vi "Normalized CC IMAQ.vi"(0 "Template U16":T1, 7 "A U16":T1, 11 "Error In":errorcluster) -> (4 "normxcorr2":dbl[][](array[numeric]), 15 "Error Out":errorcluster)   [LabVIEW 2020]
uses:
  <vilib>/vision/Image Controls.llb/IMAQ Image.ctl
  <vilib>/Analysis/2dsp.llb/2D Cross Correlation (CDB).vi
  <vilib>/Analysis/NI_AALPro.lvlib
  <vilib>/Analysis/NI_AALBase.lvlib
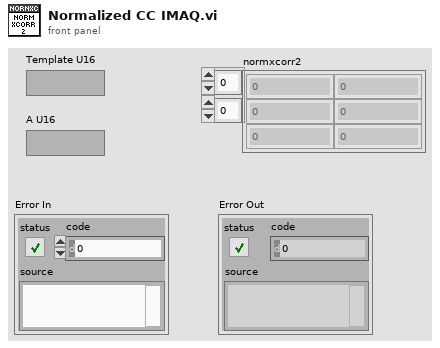
[diagram p1: front panel]
types:
  T1 = typedef "IMAQ Image.ctl" = refnum<image>
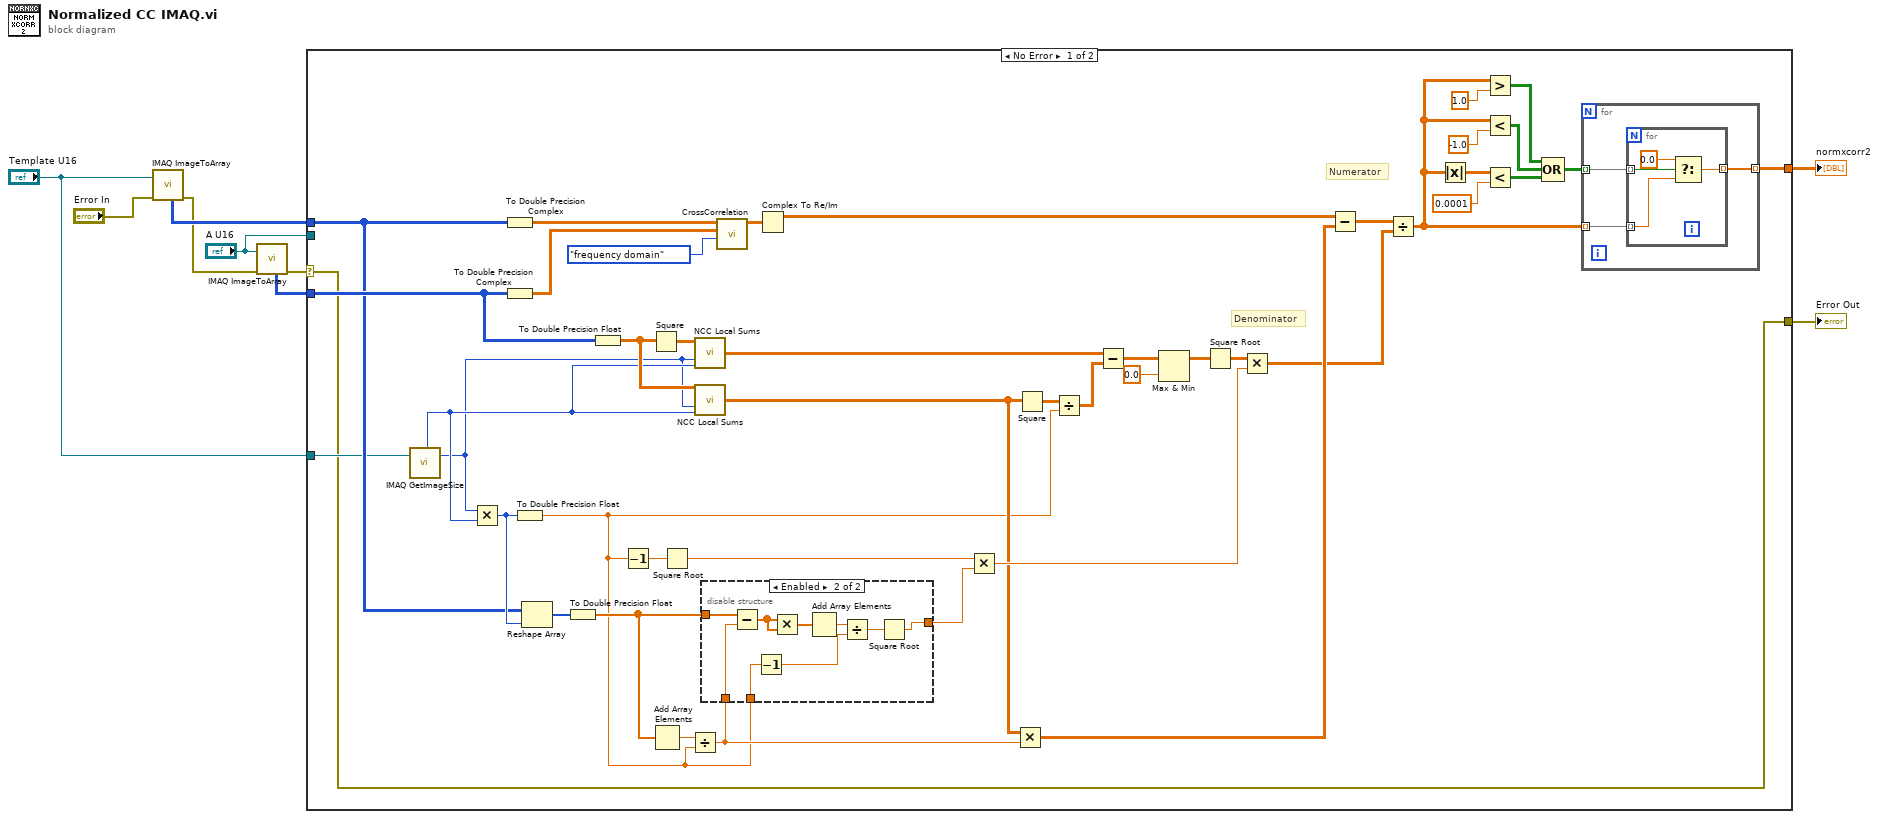
[diagram p0: block diagram]
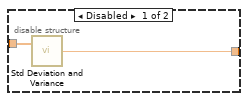
[diagram p2: hidden frame]
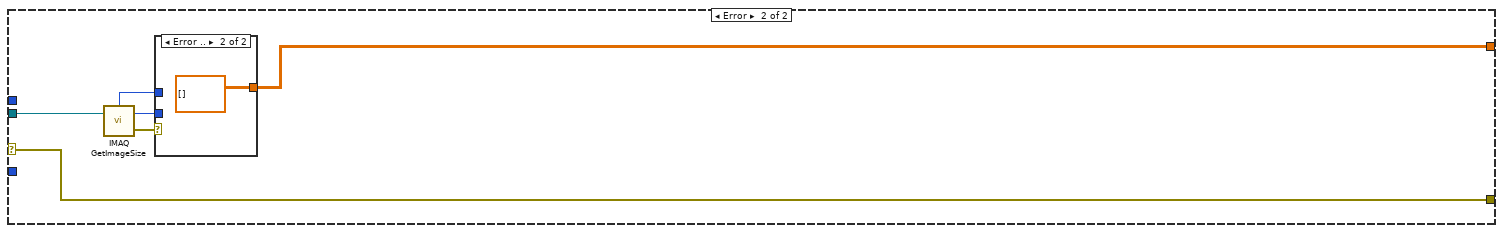
[diagram p3: hidden frame]
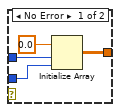
[diagram p4: hidden frame]
diagram:
  n1 = call "IMAQ ImageToArray"("error in (no error)"="Error In", "Image"="Template U16") -> ("Image Pixels (U16)"=w7:u16[][], "error out"=w4:errorcluster)  [unwired: 2 in, 3 out]
  n2 = call "IMAQ ImageToArray"("error in (no error)"=w4, "Image"="A U16") -> ("Image Pixels (U16)"=w8:u16[][], "error out"=w3:errorcluster)  [unwired: 2 in, 3 out]
  n3 = case shown="No Error" w3 {
    selector: w3 -> [w12 w72]
    tunnel: [w23 w74] -> w9
    tunnel: w8 -> [w15 _]
    tunnel: w7 -> [w14 _]
    tunnel: "Template U16" -> [w13 _]
    tunnel: "A U16" -> [_ w77]
    tunnel: [w12 w72] -> w1
    frame No Error {
      # "Denominator"
      # "Numerator"
      n4 = call "IMAQ GetImageSize"("Image"=w13) -> ("Y Resolution"=w10:i32, "X Resolution"=w11:i32)  [unwired: 3 in, 1 out]
      n5 = Multiply(x=w10, y=w11) -> (x*y=w40:i32)
      n6 = To Double Precision Complex(1:w14) -> (0:w52:cdb[][])
      n7 = To Double Precision Complex(1:w15) -> (0:w51:cdb[][])
      n8 = To Double Precision Float(number=w40) -> (double precision float=w26:dbl)
      n9 = Reshape Array(w14, w40) -> (w39:u16[])
      n10 = To Double Precision Float(number=w39) -> (double precision float=w34:dbl[])
      n11 = To Double Precision Float(number=w15) -> (double precision float=w48:dbl[][])
      n12 = Decrement(x=w26) -> (x-1=w41:dbl)
      n13 = Square(x=w48) -> (x^2=w49:dbl[][])
      n14 = Add Array Elements(numeric array=w34) -> (sum=w33:dbl)
      n15 = Square Root(x=w41) -> (sqrt(x)=w38:dbl)
      n16 = Divide(x=w33, y=w26) -> (x/y=w27:dbl)
      n17 = call "NCC Local Sums.vi"("Input Array"=w49, "Row Pad"=w10, "Col Pad"=w11) -> ("Local Sum"=w47:dbl[][])  [unwired: 12 in]
      n18 = call "NCC Local Sums.vi"("Input Array"=w48, "Row Pad"=w10, "Col Pad"=w11) -> ("Local Sum"=w32:dbl[][])  [unwired: 12 in]
      n19 = disable-structure shown="Enabled" {
        disable-tunnel: w34 -> [w62 w71]
        disable-tunnel: [w61 w63] -> w28
        disable-tunnel: w27 -> [_ w70]
        disable-tunnel: w26 -> [_ w66]
        frame Disabled {
          n20 = call <vilib>:"Std Deviation and Variance.vi"("X"=w62) -> ("standard deviation"=w61:dbl)  [unwired: 1 in, 2 out]
        }
        frame Enabled {
          n21 = Subtract(x=w71, y=w70) -> (x-y=w69:dbl[])
          n22 = Decrement(x=w66) -> (x-1=w65:dbl)
          n23 = Multiply(x=w69, y=w69) -> (x*y=w68:dbl[])
          n24 = Add Array Elements(numeric array=w68) -> (sum=w67:dbl)
          n25 = Divide(x=w67, y=w65) -> (x/y=w64:dbl)
          n26 = Square Root(x=w64) -> (sqrt(x)=w63:dbl)
        }
      }
      n27 = call-poly <vilib>:"CrossCorrelation.vi"("algorithm"=enum32{"direct", "frequency domain"}."frequency domain", "Y"=w51, "X"=w52) -> ("Rxy"=w50:cdb[][])  [unwired: 7 in, 1 out]
      n28 = Complex To Re/Im(x + iy=w50) -> (x=w35:dbl[][])  [unwired: 1 out]
      n29 = Multiply(x=w38, y=w28) -> (x*y=w36:dbl)
      n30 = Multiply(x=w32, y=w27) -> (x*y=w31:dbl[][])
      n31 = Square(x=w32) -> (x^2=w46:dbl[][])
      n32 = Divide(x=w46, y=w26) -> (x/y=w45:dbl[][])
      n33 = Subtract(x=w47, y=w45) -> (x-y=w43:dbl[][])
      n34 = Max & Min(x=w43, y=0.0) -> (max(x,y)=w42:dbl[][])  [unwired: 1 out]
      n35 = Square Root(x=w42) -> (sqrt(x)=w37:dbl[][])
      n36 = Multiply(x=w37, y=w36) -> (x*y=w29:dbl[][])
      n37 = Subtract(x=w35, y=w31) -> (x-y=w30:dbl[][])
      n38 = Divide(x=w30, y=w29) -> (x/y=w21:dbl[][])
      n39 = Absolute Value(x=w21) -> (abs(x)=w25:dbl[][])
      n40 = Greater?(x=w21, y=1.0) -> (0:w17:bool[][])
      n41 = Less?(x=w21, y=-1.0) -> (x < y?=w18:bool[][])
      n42 = Less?(x=w25, y=0.0001) -> (x < y?=w19:bool[][])
      n43 = Compound Arithmetic op=OR(w17, w18, w19) -> (w16:bool[][])
      n44 = for {
        tunnel: w21 -> [w56] mode=indexing
        tunnel: w16 -> [w55] mode=indexing
        tunnel: [w54] -> w23 mode=indexing
        n45 = for {
          tunnel: w56 -> [w59] mode=indexing
          tunnel: w55 -> [w60] mode=indexing
          tunnel: [w57] -> w54 mode=indexing
          n46 = Select(t=0.0, s=w60, f=w59) -> (s? t:f=w57:dbl)
        }
      }
    }
    frame Error {
      n47 = call "IMAQ GetImageSize"("Image"=w77) -> ("Y Resolution"=w76:i32, "X Resolution"=w75:i32, "error out"=w73:errorcluster)  [unwired: 3 in]
      n48 = case shown="Error .." w73 {
        tunnel: w76 -> [w80 _]
        tunnel: w75 -> [w81 _]
        tunnel: [w79 dbl[][] []] -> w74
        frame No Error {
          n49 = Initialize Array(0.0 ("element"), w81, w80) -> (w79:dbl[][])
        }
        frame Error {
        }
      }
    }
  }
  "normxcorr2" <- w9
  "Error Out" <- w1
